vi "compound aeithmetic.vi"() -> ()   [LabVIEW 2019]
panel:
  out "Result":bool
  in  "Boolean 1":bool=TRUE
  in  "Boolean 4":bool=TRUE
  in  "Boolean 3":bool=TRUE
  in  "Boolean 2":bool=TRUE
  out "result":dbl
  in  "Numeric 5":dbl=1.0
  in  "Numeric 4":dbl=2.0
  in  "Numeric 3":dbl=3.0
  in  "Numeric 2":dbl=4.0
  in  "Numeric1":dbl=5.0
  # "Compound Arithmetic"
  # "1) For addition and multiplication"
  # "2) For AND, OR & XOR"
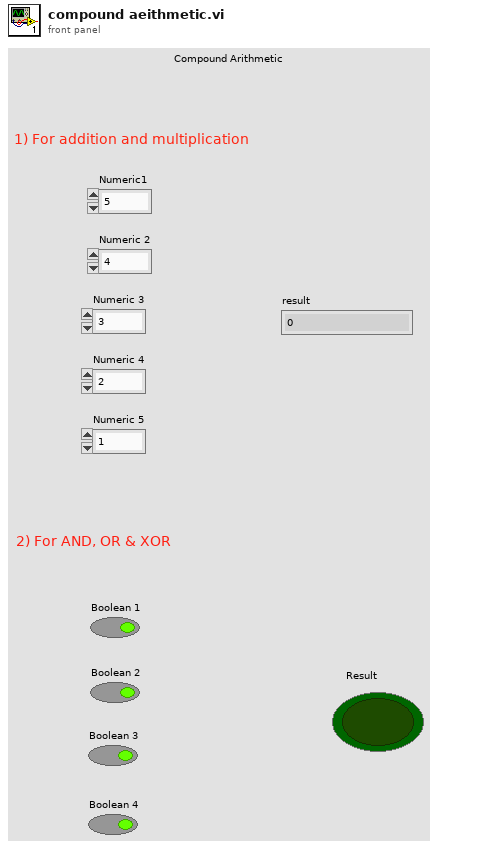
[diagram p1: front panel]
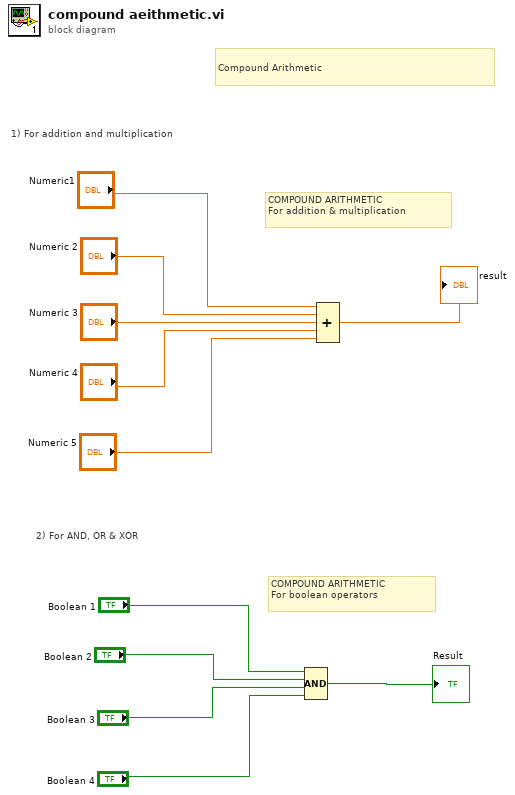
[diagram p0: block diagram]
diagram:
  # "COMPOUND ARITHMETIC \nFor addition & multiplication"
  # "COMPOUND ARITHMETIC \nFor boolean operators"
  # "1) For addition and multiplication"
  # "2) For AND, OR & XOR"
  # "Compound Arithmetic"
  n1 = Compound Arithmetic op=AND("Boolean 1", "Boolean 2", "Boolean 3", "Boolean 4") -> (→"Result":bool)
  n2 = Compound Arithmetic op=ADD("Numeric1", "Numeric 2", "Numeric 3", "Numeric 4", "Numeric 5") -> (→"result":dbl)
